vi "RunningEdgeCount.vi"(6 "Prior Lows":u8=10, 7 "Reset Count? (F)":bool, 10 "Input":bool) -> (1 "Rising Edge?":bool, 2 "Count":u32)   [LabVIEW 2018]
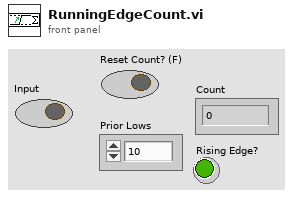
[diagram p1: front panel]
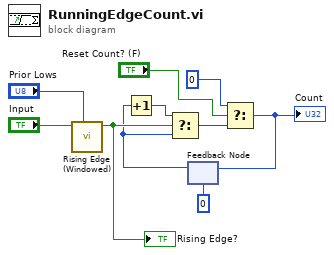
[diagram p0: block diagram]
diagram:
  n1 = call "Rising Edge (Windowed).vi"("Prior Lows"="Prior Lows", "Input"="Input") -> ("Rising Edge?"=w9:bool)  [unwired: 9 in]
  "Rising Edge?" <- w9
  n2 = feedback #1(u32 0) -> (w8:u32)
  n3 = Increment(x=w8) -> (x+1=w7:u32)
  n4 = Select(t=w7, s=w9, f=w8) -> (s? t:f=w6:u32)
  n5 = Select(t=u32 0, s="Reset Count? (F)", f=w6) -> (s? t:f=w3:u32)
  "Count" <- w3
  n6 = feedback-in #1(w3) -> ()
